vi "Car Control.vi"(7 "Reset":bool, 10 "Car Info":T2 {"Heading" format="%.1f"; "Y" format="%.3f"; "X" format="%.3f"; "Speed" format="%.2f"}, 11 "Ranges":T1 {"Rear" format="%.3f"; "Front" format="%.3f"}) -> (2 "Throttle (0 to 1)":sgl, 3 "Steering (-1 to 1)":sgl)   [LabVIEW 2020]
uses:
  FormulaLV-Common/Car Info.ctl
  FormulaLV-Common/Ranges.ctl
  FormulaLV-Common/FormulaG-Common.lvlib
panel:
  in  "Throttle":sgl(slide)=0.16083916 scale=0.0..1.0
  in  "Steering Sensitivity":sgl(slide)=0.5244755 scale=0.0..1.0
  # "Additional controls and indicators can be added to this VI to help with tuning control parameters and providing debugging info. This VI can be left open while the game runs so you can tweak its operation.\n\nEnsure you remember to set control value defaults by selecting them and choosing Make Selected Values Default in the Edit menu so parameters persist after closing the project, or you should change them to block diagram constants once they're set appropriately."
  # "** DO NOT CHANGE THE CONNECTOR PANE OF THIS VI **\nThese controls and indicators are for the standard inputs and outputs for this VI; trying to change these controls has no effect as they're set by the engine."
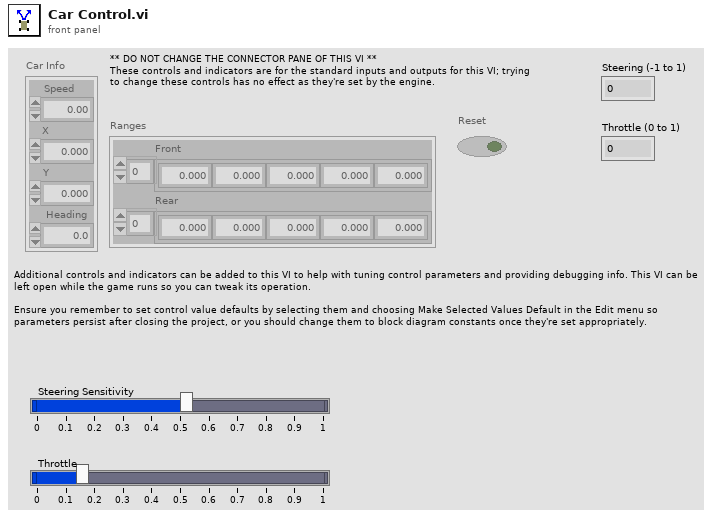
[diagram p1: front panel]
types:
  T1 = typedef "FormulaG-Common.lvlib/Ranges.ctl" = cluster{"Front":sgl[], "Rear":sgl[]}
  T2 = typedef "FormulaG-Common.lvlib/Car Info.ctl" = cluster{"Speed":sgl, "X":sgl, "Y":sgl, "Heading":sgl}
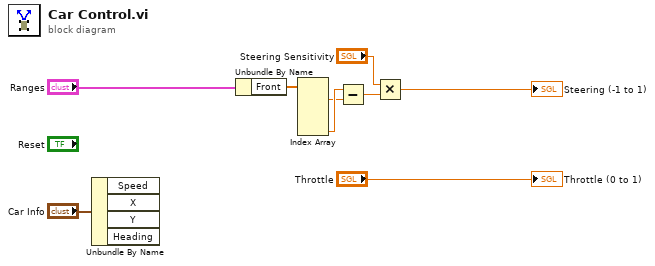
[diagram p0: block diagram]
diagram:
  n1 = Unbundle By Name("Car Info") -> ()  [unwired: 4 out]
  n2 = Unbundle By Name("Ranges") -> ("Front"=w8:sgl[])
  n3 = Index Array(array=w8) -> (element #1=w6:sgl, element #5=w7:sgl)  [unwired: 5 in, 3 out]
  n4 = Subtract(x=w7, y=w6) -> (x-y=w5:sgl)
  n5 = Multiply(x="Steering Sensitivity", y=w5) -> (x*y=→"Steering (-1 to 1)":sgl)
  "Throttle (0 to 1)" <- "Throttle"
